vi "Euler_ang2quat (SubVI).vi"(11 "Euler Angles [deg]":cluster{"phi":dbl, "theta":dbl, "psi":dbl}) -> (3 "Quaternions":dbl[](array[numeric]))   [LabVIEW 2011]
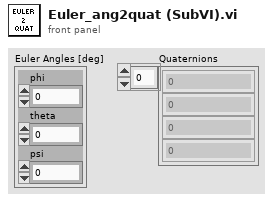
[diagram p1: front panel]
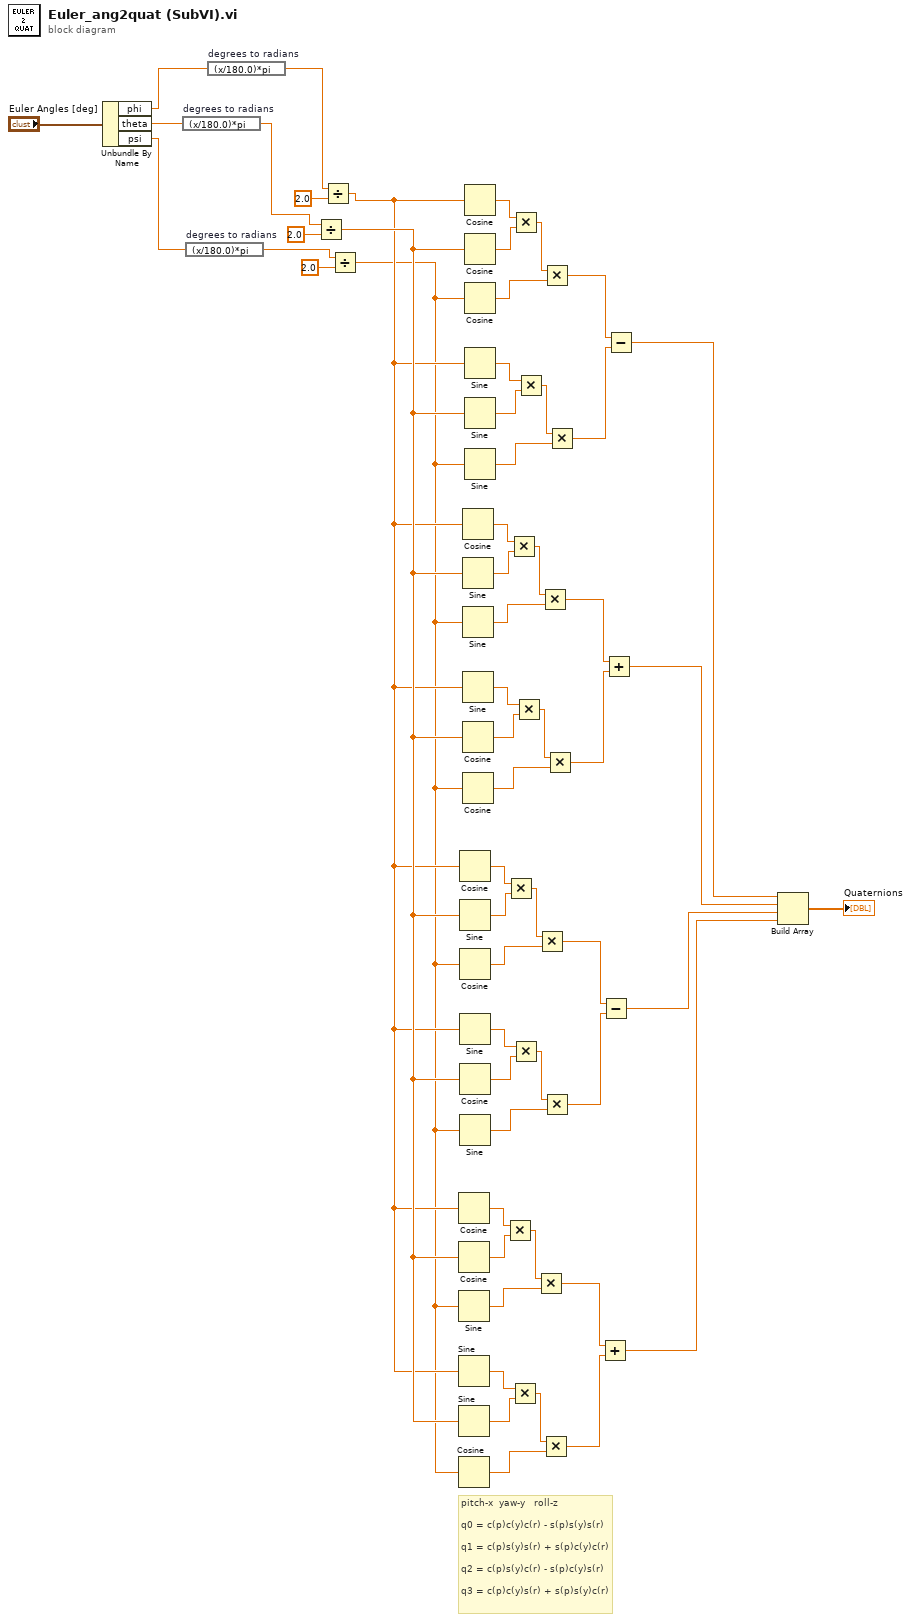
[diagram p0: block diagram]
diagram:
  # "pitch-x  yaw-y   roll-z\n\nq0 = c(p)c(y)c(r) - s(p)s(y)s(r)\n\nq1 = c(p)s(y)s(r) + s(p)c(y)c(r)\n\nq2 = c(p)s(y)c(r) - s(p)c(y)s(r)\n\nq3 = c(p)c(y)s(r) + s(p)s(y)c(r)"
  n1 = Unbundle By Name("Euler Angles [deg]") -> ("phi"=w6:dbl, "theta"=w4:dbl, "psi"=w2:dbl)
  n2 = expression code="(x/180.0)*pi" "degrees to radians"(w4) -> (w3:dbl)
  n3 = expression code="(x/180.0)*pi" "degrees to radians"(w2) -> (w1:dbl)
  n4 = expression code="(x/180.0)*pi" "degrees to radians"(w6) -> (w5:dbl)
  n5 = Divide(x=w3, y=2.0) -> (x/y=w58:dbl)
  n6 = Divide(x=w5, y=2.0) -> (x/y=w56:dbl)
  n7 = Divide(x=w1, y=2.0) -> (x/y=w8:dbl)
  n8 = Cosine(x=w56) -> (cos(x)=w49:dbl)
  n9 = Cosine(x=w58) -> (cos(x)=w48:dbl)
  n10 = Sine(x=w8) -> (sin(x)=w46:dbl)
  n11 = Sine(x=w56) -> (sin(x)=w44:dbl)
  n12 = Sine(x=w58) -> (sin(x)=w43:dbl)
  n13 = Cosine(x=w8) -> (cos(x)=w42:dbl)
  n14 = Cosine(x=w56) -> (cos(x)=w30:dbl)
  n15 = Sine(x=w58) -> (sin(x)=w31:dbl)
  n16 = Cosine(x=w8) -> (cos(x)=w33:dbl)
  n17 = Sine(x=w56) -> (sin(x)=w35:dbl)
  n18 = Cosine(x=w58) -> (cos(x)=w36:dbl)
  n19 = Sine(x=w8) -> (sin(x)=w37:dbl)
  n20 = Cosine(x=w56) -> (cos(x)=w29:dbl)
  n21 = Sine(x=w58) -> (sin(x)=w28:dbl)
  n22 = Sine(x=w8) -> (sin(x)=w26:dbl)
  n23 = Sine(x=w56) -> (sin(x)=w24:dbl)
  n24 = Cosine(x=w58) -> (cos(x)=w23:dbl)
  n25 = Cosine(x=w8) -> (cos(x)=w22:dbl)
  n26 = Cosine(x=w56) -> (cos(x)=w10:dbl)
  n27 = Cosine(x=w58) -> (cos(x)=w11:dbl)
  n28 = Cosine(x=w8) -> (cos(x)=w13:dbl)
  n29 = Sine(x=w56) -> (sin(x)=w15:dbl)
  n30 = Sine(x=w58) -> (sin(x)=w16:dbl)
  n31 = Sine(x=w8) -> (sin(x)=w17:dbl)
  n32 = Multiply(x=w49, y=w48) -> (x*y=w47:dbl)
  n33 = Multiply(x=w30, y=w31) -> (x*y=w32:dbl)
  n34 = Multiply(x=w29, y=w28) -> (x*y=w27:dbl)
  n35 = Multiply(x=w44, y=w43) -> (x*y=w45:dbl)
  n36 = Multiply(x=w10, y=w11) -> (x*y=w12:dbl)
  n37 = Multiply(x=w35, y=w36) -> (x*y=w34:dbl)
  n38 = Multiply(x=w24, y=w23) -> (x*y=w25:dbl)
  n39 = Multiply(x=w15, y=w16) -> (x*y=w14:dbl)
  n40 = Multiply(x=w47, y=w46) -> (x*y=w41:dbl)
  n41 = Multiply(x=w32, y=w33) -> (x*y=w38:dbl)
  n42 = Multiply(x=w27, y=w26) -> (x*y=w21:dbl)
  n43 = Multiply(x=w45, y=w42) -> (x*y=w40:dbl)
  n44 = Multiply(x=w12, y=w13) -> (x*y=w18:dbl)
  n45 = Multiply(x=w34, y=w37) -> (x*y=w39:dbl)
  n46 = Multiply(x=w25, y=w22) -> (x*y=w20:dbl)
  n47 = Multiply(x=w14, y=w17) -> (x*y=w19:dbl)
  n48 = Add(x=w41, y=w40) -> (x+y=w53:dbl)
  n49 = Subtract(x=w38, y=w39) -> (x-y=w52:dbl)
  n50 = Add(x=w21, y=w20) -> (x+y=w51:dbl)
  n51 = Subtract(x=w18, y=w19) -> (x-y=w50:dbl)
  n52 = Build Array(w50, w51, w52, w53) -> (→"Quaternions":dbl[])
